vi "Untitled 7.vi"() -> ()   [LabVIEW 2024]
panel:
  out "appended path":path
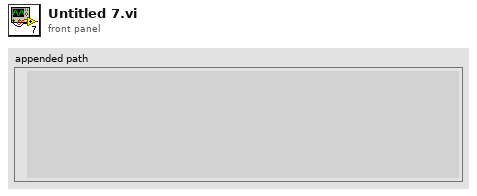
[diagram p1: front panel]
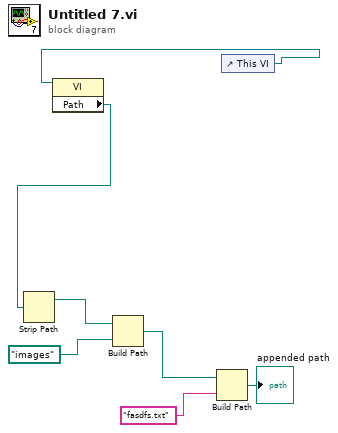
[diagram p0: block diagram]
diagram:
  n1 = control-ref of="This VI"() -> (w6:refnum<vi>)
  n2 = property class="VI"(reference=w6) -> ("Path"=w5:path)  [unwired: 1 in, 2 out]
  n3 = Strip Path(path=w5) -> (stripped path=w4:path)  [unwired: 1 out]
  n4 = Build Path(base path=w4, name or relative path=path "images") -> (appended path=w3:path)
  n5 = Build Path(base path=w3, name or relative path="fasdfs.txt" ("initial string")) -> (appended path=→"appended path":path)
